vi "Get GObject.vi"(8 "error in (no error)":errorcluster, 10 "GObject UID":string, 11 "VI Data in":refnum<class "VI Data.lvclass">) -> (0 "error out":errorcluster, 1 "GObject":refnum<class "GObject.lvclass">, 2 "found":bool, 3 "VI Data out":refnum<class "VI Data.lvclass">)   [LabVIEW 2013, in "SET Project Data.lvlib" / "VI Data.lvclass"]
uses:
  VI Data.lvclass
  Control Classes/GObject/GObject.lvclass
  VI Data.lvclass/VI Data.ctl
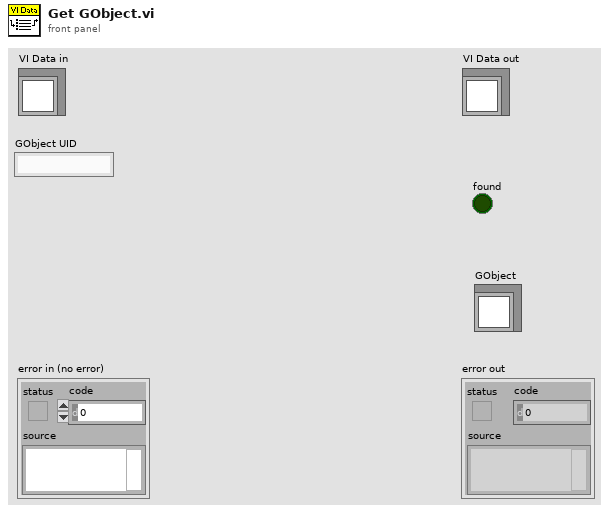
[diagram p1: front panel]
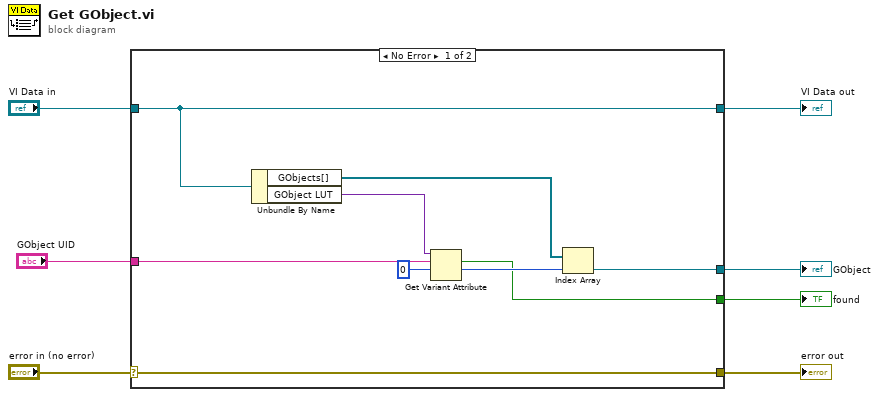
[diagram p0: block diagram]
diagram:
  n1 = case shown="No Error" "error in (no error)" {
    selector: "error in (no error)" -> [w16 w18]
    tunnel: [w16 w18] -> w6
    tunnel: [w15 w17] -> w4
    tunnel: "VI Data in" -> [w15 w17]
    tunnel: "GObject UID" -> [w13 _]
    tunnel: [w9 _] -> w2
    tunnel: [w8 _] -> w1
    frame No Error {
      n2 = Unbundle By Name(w15) -> ("GObjects[]"=w11:refnum<class "GObject.lvclass">[], "GObject LUT"=w14:variant)
      n3 = Get Variant Attribute(Variant=w14, name=w13, default value (empty Variant)=0) -> (found=w9:bool, value=w10:i32)  [unwired: 1 in, 2 out]
      n4 = Index Array(array=w11, index=w10) -> (element=w8:refnum<class "GObject.lvclass">)
    }
    frame Error {
    }
  }
  "error out" <- w6
  "VI Data out" <- w4
  "found" <- w2
  "GObject" <- w1
